vi "（自研）一通知器控制多条件分支与多通知器对一通讯.vi"() -> ()   [LabVIEW 2016]
panel:
  out "通知器名":string
  out "通知":string[](array[string])
  in  "邓三弟":bool
  in  "邓二哥":bool
  in  "邓大大":bool
  in  "停止":bool
  in  "字符串":string
  in  "簇":cluster{"通知器":string}
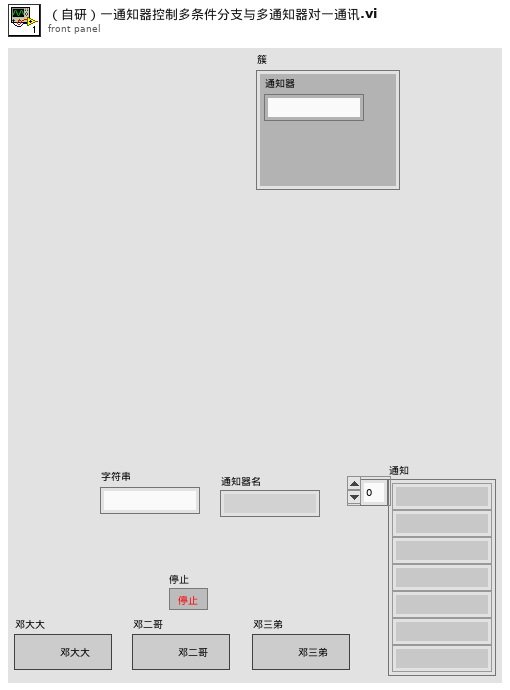
[diagram p1: front panel]
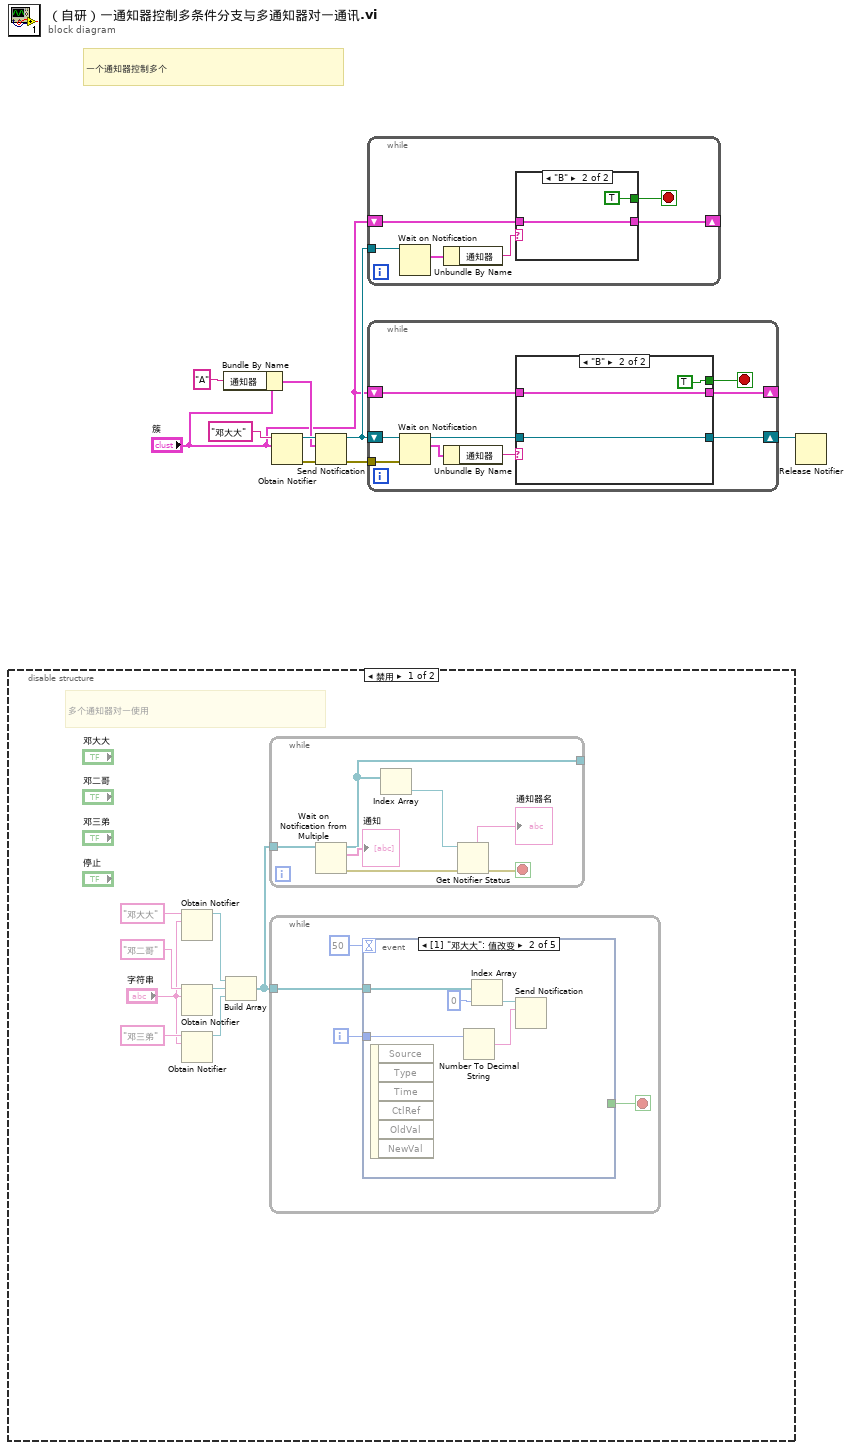
[diagram p0: block diagram]
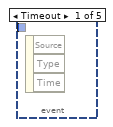
[diagram p2: hidden frame]
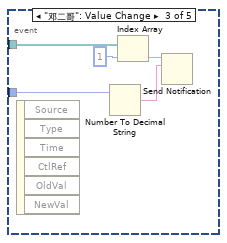
[diagram p3: hidden frame]
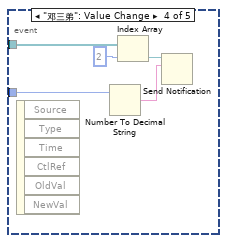
[diagram p4: hidden frame]
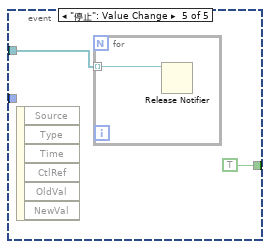
[diagram p5: hidden frame]
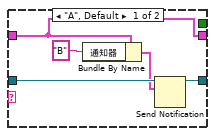
[diagram p8: hidden frame]
diagram:
  # "一个通知器控制多个"
  n1 = disable-structure shown="禁用" {
    frame Disabled {
      # "多个通知器对一使用"
      n2 = Obtain Notifier(name (unnamed)="邓大大" ("名称（未命名）"), notification data type="字符串") -> (notifier out=w13:refnum<notifier>)  [unwired: 2 in, 2 out]
      n3 = Obtain Notifier(name (unnamed)="邓二哥" ("名称（未命名）"), notification data type="字符串") -> (notifier out=w12:refnum<notifier>)  [unwired: 2 in, 2 out]
      n4 = Obtain Notifier(name (unnamed)="邓三弟" ("名称（未命名）"), notification data type="字符串") -> (notifier out=w11:refnum<notifier>)  [unwired: 2 in, 2 out]
      n5 = Build Array(w13, w12, w11) -> (w10:refnum<notifier>[])
      n6 = while {
        tunnel: w10 -> [w46]
        tunnel: [w44] -> _
        stop <- w40 stop-if-true
        n7 = Wait on Notification from Multiple(0:w46) -> (8:w44:refnum<notifier>[], 9:→"通知":string[], 11:w41:errorcluster)  [unwired: 3 in, 1 out]
        n8 = Index Array(array=w44) -> (element=w43:refnum<notifier>)  [unwired: 1 in]
        n9 = Get Notifier Status(notifier=w43, error in (no error)=w41) -> (notifier name=→"通知器名":string, error out=w40:errorcluster)  [unwired: 3 out]
      }
      n10 = while {
        tunnel: w10 -> [w21]
        i -> [w19]
        stop <- w18 stop-if-true
        n11 = event shown="[1] \"邓大大\": 值改变" {
          selector: _ -> [_ _ _ _ _]
          dyn-events: _ -> [_ _ _ _ _]
          timeout: 50 -> [_ _ _ _ _]
          tunnel: w21 -> [_ w26 w28 w33 w38]
          tunnel: w19 -> [_ w23 w27 w32 _]
          tunnel: [_ _ _ _ TRUE] -> w18
          event Timeout {
            n12 = event-data() -> ()  [unwired: 1 in, 3 out]
          }
          event "邓大大": Value Change {
            n13 = event-data() -> ()  [unwired: 1 in, 6 out]
            n14 = Number To Decimal String(number=w23) -> (decimal integer string=w22:string)  [unwired: 1 in]
            n15 = Index Array(array=w26, index=0 ("索引")) -> (element=w24:refnum<notifier>)
            n16 = Send Notification(notification=w22, notifier=w24) -> ()  [unwired: 1 in, 2 out]
          }
          event "邓二哥": Value Change {
            n17 = event-data() -> ()  [unwired: 1 in, 6 out]
            n18 = Number To Decimal String(number=w27) -> (decimal integer string=w29:string)  [unwired: 1 in]
            n19 = Index Array(array=w28, index=1 ("索引")) -> (element=w30:refnum<notifier>)
            n20 = Send Notification(notification=w29, notifier=w30) -> ()  [unwired: 1 in, 2 out]
          }
          event "邓三弟": Value Change {
            n21 = event-data() -> ()  [unwired: 1 in, 6 out]
            n22 = Number To Decimal String(number=w32) -> (decimal integer string=w34:string)  [unwired: 1 in]
            n23 = Index Array(array=w33, index=2 ("索引")) -> (element=w35:refnum<notifier>)
            n24 = Send Notification(notification=w34, notifier=w35) -> ()  [unwired: 1 in, 2 out]
          }
          event "停止": Value Change {
            n25 = event-data() -> ()  [unwired: 1 in, 6 out]
            n26 = for {
              tunnel: w38 -> [w39] mode=indexing
              n27 = Release Notifier(notifier=w39) -> ()  [unwired: 2 in, 3 out]
            }
          }
        }
      }
    }
    frame Enabled {
    }
  }
  n28 = Bundle By Name(cluster="簇", "通知器"="A") -> (w6:cluster{"通知器":string})
  n29 = Obtain Notifier(name (unnamed)="邓大大" ("名称（未命名）"), notification data type="簇") -> (notifier out=w8:refnum<notifier>, error out=w5:errorcluster)  [unwired: 2 in, 1 out]
  n30 = Send Notification(notification=w6, notifier=w8, error in (no error)=w5) -> (notifier out=w3:refnum<notifier>, error out=w4:errorcluster)
  n31 = while {
    tunnel: w3 -> [w52]
    shift-right: [w50] -> _
    shift-left: "簇" -> [w51]
    stop <- w49 stop-if-true
    n32 = Wait on Notification(notifier=w52) -> (notification=w48:cluster{"通知器":string})  [unwired: 3 in, 3 out]
    n33 = Unbundle By Name(w48) -> ("通知器"=w47:string)
    n34 = case shown="\"B\"" w47 {
      tunnel: w51 -> [w53 w55]
      tunnel: [w53 w55] -> w50
      tunnel: [_ TRUE] -> w49
      frame "A", Default {
      }
      frame "B" {
      }
    }
  }
  n35 = while {
    shift-right: [w62] -> _
    shift-left: "簇" -> [w63]
    tunnel: w4 -> [w60]
    shift-right: [w56] -> w1
    shift-left: w3 -> [w64]
    stop <- w57 stop-if-true
    n36 = Wait on Notification(notifier=w64, error in (no error)=w60) -> (notifier out=w61:refnum<notifier>, notification=w59:cluster{"通知器":string})  [unwired: 2 in, 2 out]
    n37 = Unbundle By Name(w59) -> ("通知器"=w58:string)
    n38 = case shown="\"B\"" w58 {
      tunnel: w63 -> [w67 w72]
      tunnel: [w67 w72] -> w62
      tunnel: w61 -> [w69 w71]
      tunnel: [w68 w71] -> w56
      tunnel: [_ TRUE] -> w57
      frame "A", Default {
        n39 = Bundle By Name(cluster=w67, "通知器"="B") -> (w66:cluster{"通知器":string})
        n40 = Send Notification(notification=w66, notifier=w69) -> (notifier out=w68:refnum<notifier>)  [unwired: 1 in, 1 out]
      }
      frame "B" {
      }
    }
  }
  n41 = Release Notifier(notifier=w1) -> ()  [unwired: 2 in, 3 out]
